vi "Décomposition tableau String 1D.vi"(11 "appended array in":string[](array[string])) -> (0 "7":i32, 1 "6":i32, 2 "4":i32, 3 "3":i32, 4 "8":i32, 5 "2":i32, 6 "9":i32, 7 "1":i32)   [LabVIEW 2019]
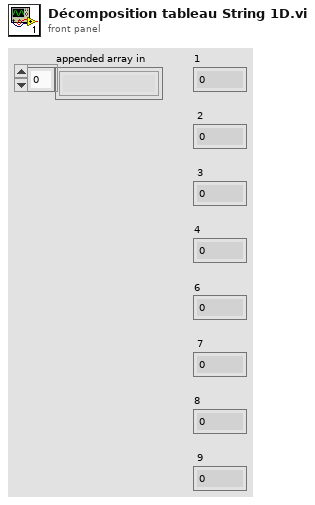
[diagram p1: front panel]
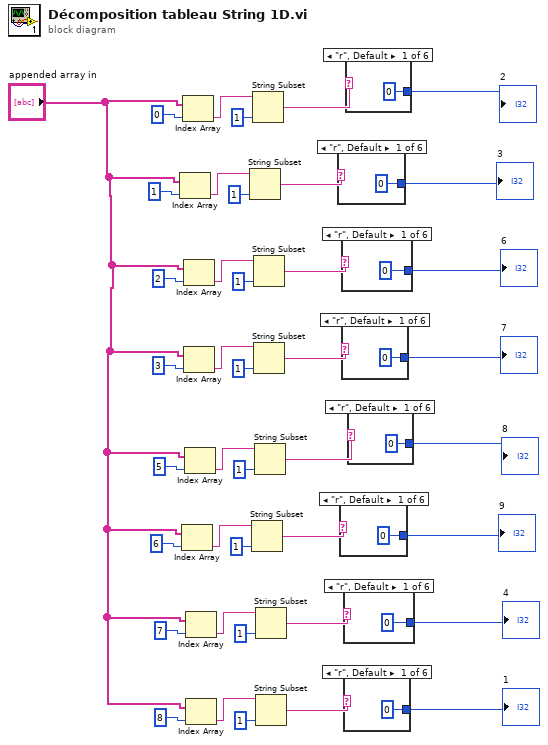
[diagram p0: block diagram]
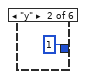
[diagram p2: hidden frame]
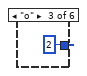
[diagram p3: hidden frame]
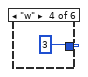
[diagram p4: hidden frame]
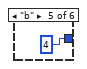
[diagram p5: hidden frame]
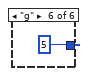
[diagram p6: hidden frame]
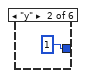
[diagram p7: hidden frame]
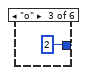
[diagram p8: hidden frame]
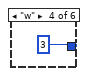
[diagram p9: hidden frame]
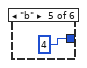
[diagram p10: hidden frame]
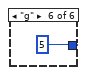
[diagram p11: hidden frame]
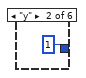
[diagram p12: hidden frame]
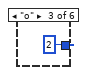
[diagram p13: hidden frame]
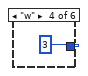
[diagram p14: hidden frame]
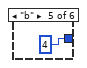
[diagram p15: hidden frame]
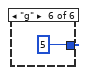
[diagram p16: hidden frame]
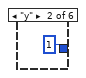
[diagram p17: hidden frame]
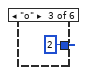
[diagram p18: hidden frame]
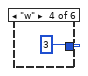
[diagram p19: hidden frame]
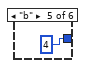
[diagram p20: hidden frame]
diagram:
  n1 = Index Array(array="appended array in", index=1) -> (element=w7:string)
  n2 = Index Array(array="appended array in", index=6) -> (element=w34:string)
  n3 = Index Array(array="appended array in", index=0) -> (element=w19:string)
  n4 = Index Array(array="appended array in", index=2) -> (element=w10:string)
  n5 = Index Array(array="appended array in", index=3) -> (element=w17:string)
  n6 = Index Array(array="appended array in", index=5) -> (element=w22:string)
  n7 = Index Array(array="appended array in", index=7) -> (element=w31:string)
  n8 = Index Array(array="appended array in", index=8) -> (element=w24:string)
  n9 = String Subset(string=w7, length (rest)=1 ("length (rest)")) -> (substring=w5:string)  [unwired: 1 in]
  n10 = String Subset(string=w34, length (rest)=1 ("length (rest)")) -> (substring=w36:string)  [unwired: 1 in]
  n11 = String Subset(string=w19, length (rest)=1 ("length (rest)")) -> (substring=w20:string)  [unwired: 1 in]
  n12 = String Subset(string=w10, length (rest)=1 ("length (rest)")) -> (substring=w12:string)  [unwired: 1 in]
  n13 = String Subset(string=w17, length (rest)=1 ("length (rest)")) -> (substring=w15:string)  [unwired: 1 in]
  n14 = String Subset(string=w22, length (rest)=1 ("length (rest)")) -> (substring=w21:string)  [unwired: 1 in]
  n15 = String Subset(string=w31, length (rest)=1 ("length (rest)")) -> (substring=w29:string)  [unwired: 1 in]
  n16 = String Subset(string=w24, length (rest)=1 ("length (rest)")) -> (substring=w26:string)  [unwired: 1 in]
  n17 = case shown="\"r\", Default" w5 {
    tunnel: [0 1 2 3 4 5] -> w4
    frame "r", Default {
    }
    frame "y" {
    }
    frame "o" {
    }
    frame "w" {
    }
    frame "b" {
    }
    frame "g" {
    }
  }
  "3" <- w4
  n18 = case shown="\"r\", Default" w36 {
    tunnel: [0 1 2 3 4 5] -> w37
    frame "r", Default {
    }
    frame "y" {
    }
    frame "o" {
    }
    frame "w" {
    }
    frame "b" {
    }
    frame "g" {
    }
  }
  "9" <- w37
  n19 = case shown="\"r\", Default" w12 {
    tunnel: [0 1 2 3 4 5] -> w13
    frame "r", Default {
    }
    frame "y" {
    }
    frame "o" {
    }
    frame "w" {
    }
    frame "b" {
    }
    frame "g" {
    }
  }
  "6" <- w13
  n20 = case shown="\"r\", Default" w15 {
    tunnel: [0 1 2 3 4 5] -> w14
    frame "r", Default {
    }
    frame "y" {
    }
    frame "o" {
    }
    frame "w" {
    }
    frame "b" {
    }
    frame "g" {
    }
  }
  "7" <- w14
  n21 = case shown="\"r\", Default" w29 {
    tunnel: [0 1 2 3 4 5] -> w28
    frame "r", Default {
    }
    frame "y" {
    }
    frame "o" {
    }
    frame "w" {
    }
    frame "b" {
    }
    frame "g" {
    }
  }
  "4" <- w28
  n22 = case shown="\"r\", Default" w26 {
    tunnel: [0 1 2 3 4 5] -> w27
    frame "r", Default {
    }
    frame "y" {
    }
    frame "o" {
    }
    frame "w" {
    }
    frame "b" {
    }
    frame "g" {
    }
  }
  "1" <- w27
  n23 = case shown="\"r\", Default" w20 {
    tunnel: [0 1 2 3 4 5] -> w3
    frame "r", Default {
    }
    frame "y" {
    }
    frame "o" {
    }
    frame "w" {
    }
    frame "b" {
    }
    frame "g" {
    }
  }
  "2" <- w3
  n24 = case shown="\"r\", Default" w21 {
    tunnel: [0 1 2 3 4 5] -> w38
    frame "r", Default {
    }
    frame "y" {
    }
    frame "o" {
    }
    frame "w" {
    }
    frame "b" {
    }
    frame "g" {
    }
  }
  "8" <- w38
